vi "数据DIY样例程序.vi"() -> ()   [LabVIEW 2020]
panel:
  out "自动路径":cluster{"路径点名":string, "路径插补":string}[](array[cluster])
  out "坐标点名":string[][](table) caption="output array"
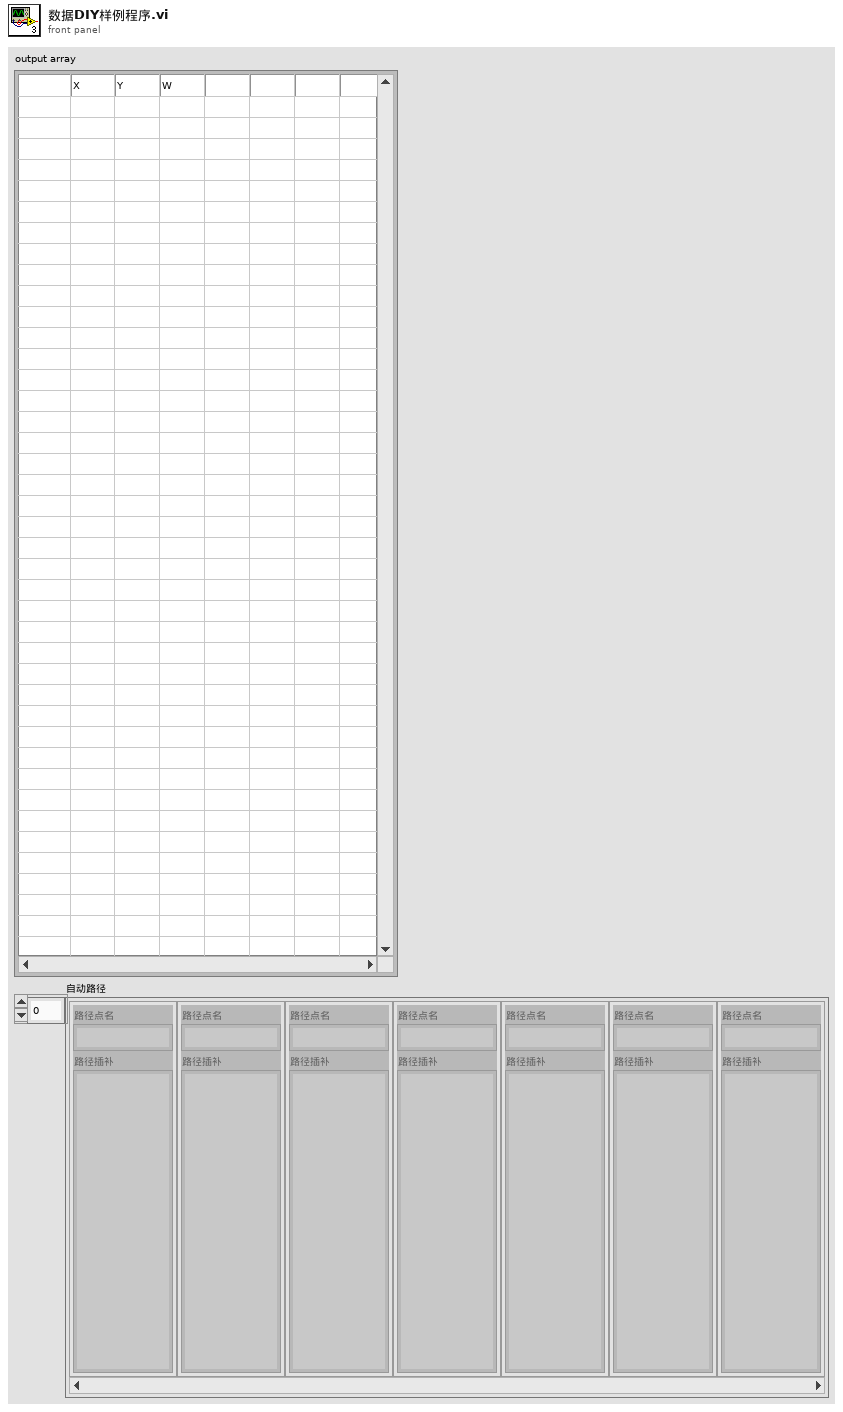
[diagram p1: front panel]
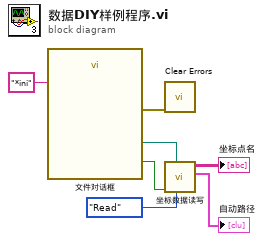
[diagram p0: block diagram]
diagram:
  n1 = call "文件对话框"("pattern (all files)"="*ini") -> ("selected path"=w7:path, "exists"=w4:bool, "error out"=w5:errorcluster)  [unwired: 11 in, 1 out]
  n2 = call <vilib>:"Clear Errors.vi"("error in (no error)"=w5) -> ()  [unwired: 5 in, 2 out]
  n3 = call "坐标数据读写.vi"("model"=enum16{"Read", "Write", "Delete"}."Read", "Path"=w7, "布尔"=w4) -> ("自动路径 out"=→"自动路径":cluster{"路径点名":string, "路径插补":string}[], "坐标点名 2"=→"坐标点名":string[][])  [unwired: 5 in, 2 out]
